vi "VersaLaseGUI_ForMain.vi"() -> ()   [LabVIEW 2014]
uses:
  C:/Users/Avogadro/Desktop/VersaUSB/VersaUSB.dll
  VersaUSB.dll
panel:
  out "ne":i32
  out "e":i32
  in  "Blu Pow":dbl(slide) scale=0.0..100.0
  in  "Grn Pow":dbl(slide) scale=0.0..40.0
  in  "Blu On":bool
  in  "Grn On":bool
  out "Blu Temp":dbl
  out "Grn Temp":dbl
  in  "Red Pow":dbl(slide) scale=0.0..100.0
  in  "Red On":bool
  out "Red Temp":dbl
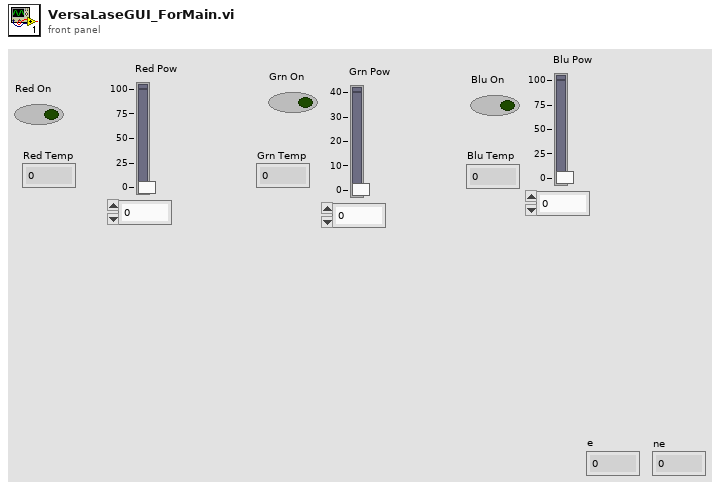
[diagram p1: front panel]
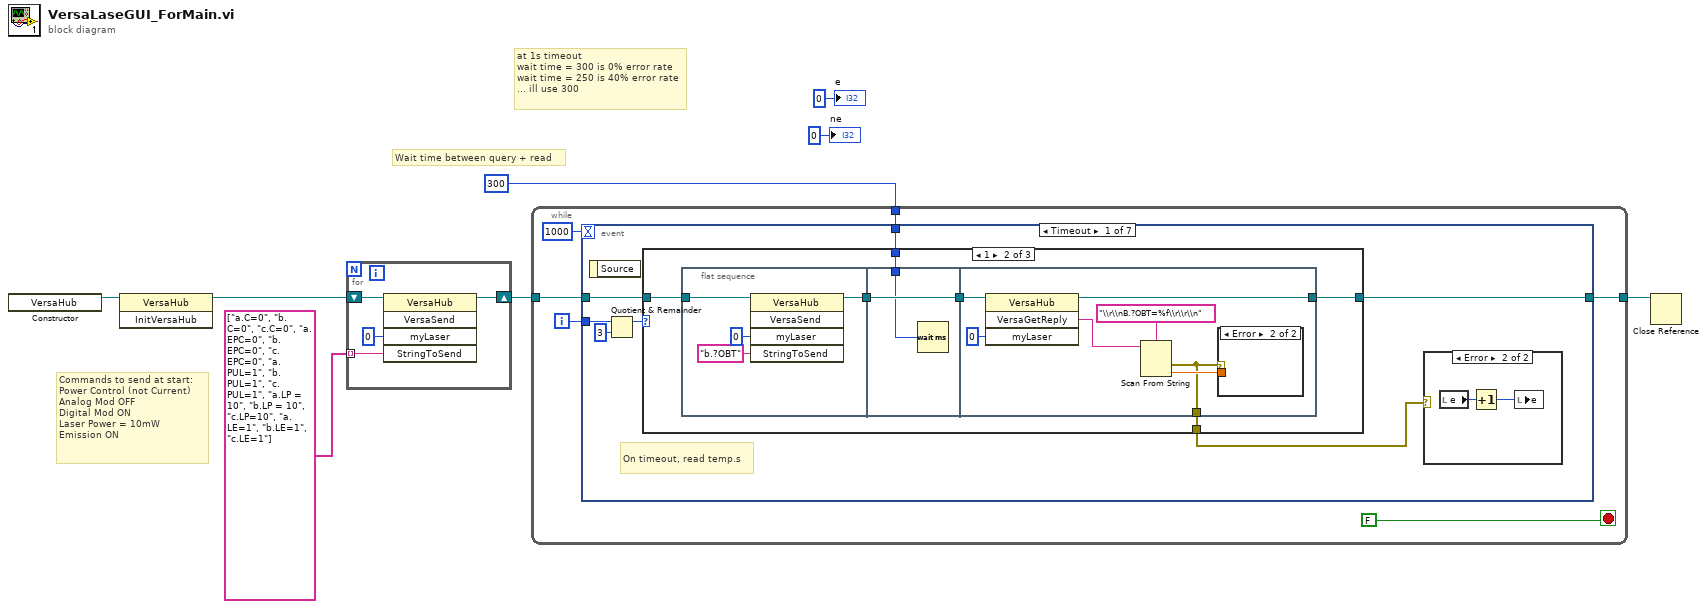
[diagram p0: block diagram]
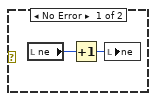
[diagram p2: hidden frame]
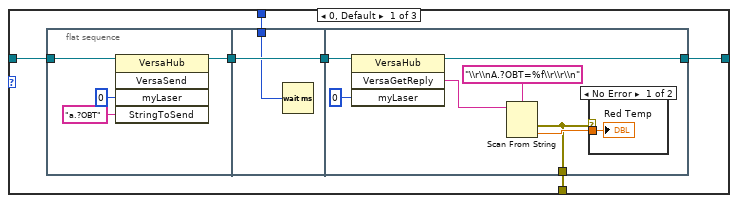
[diagram p3: hidden frame]
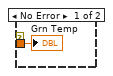
[diagram p5: hidden frame]
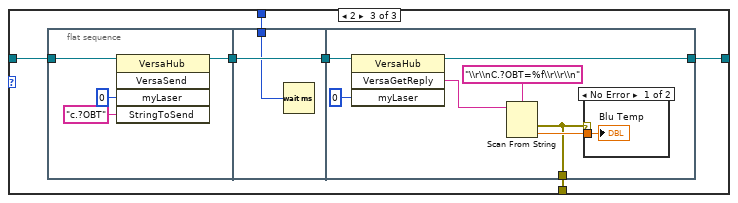
[diagram p6: hidden frame]
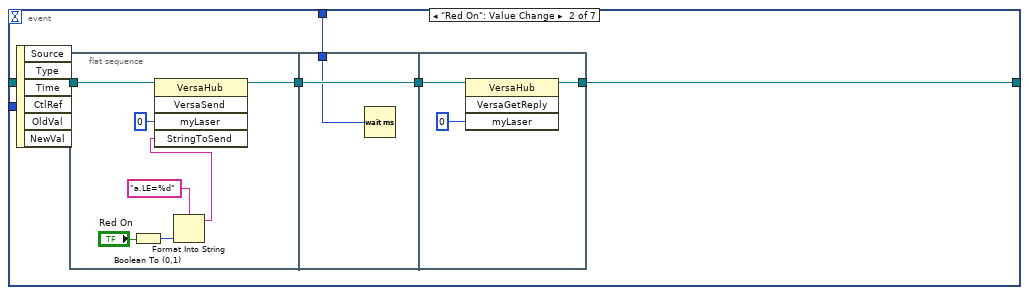
[diagram p8: hidden frame]
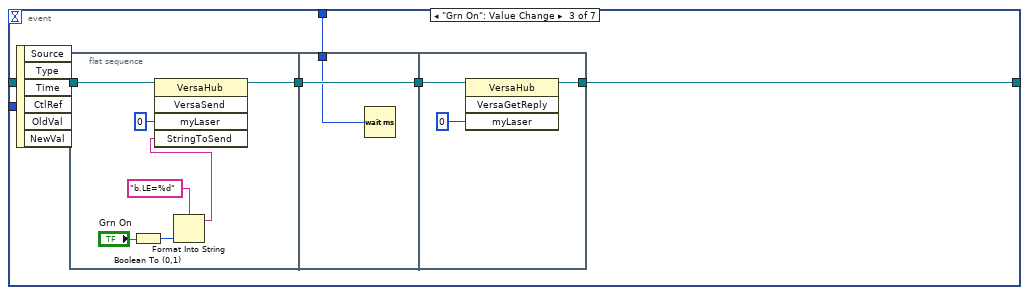
[diagram p9: hidden frame]
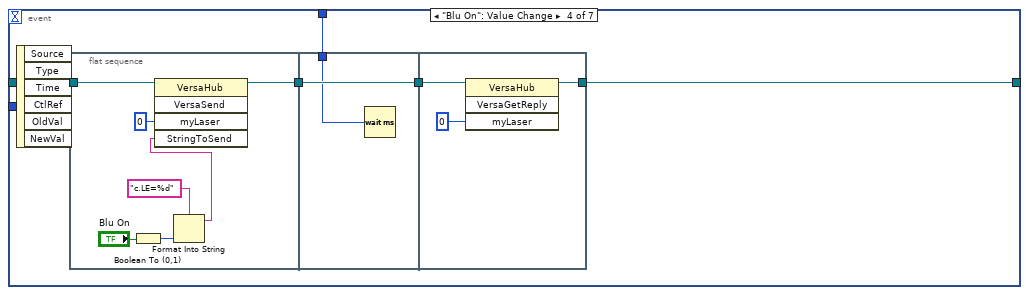
[diagram p10: hidden frame]
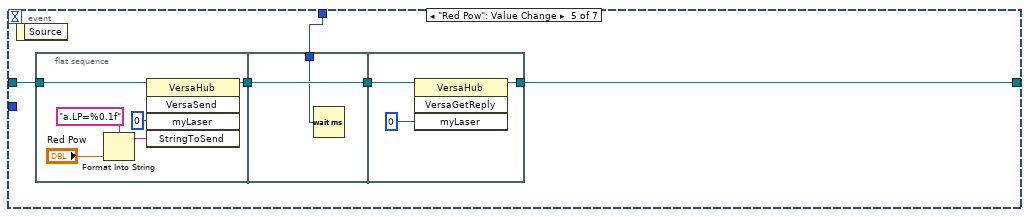
[diagram p11: hidden frame]
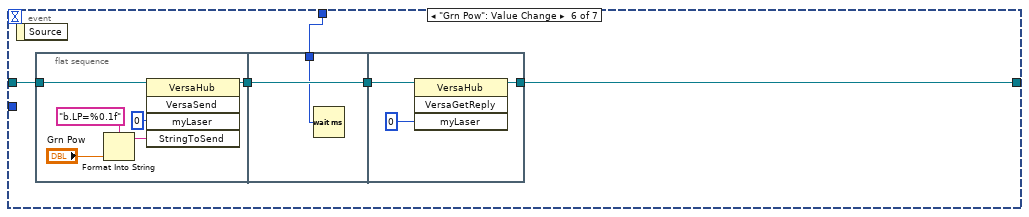
[diagram p12: hidden frame]
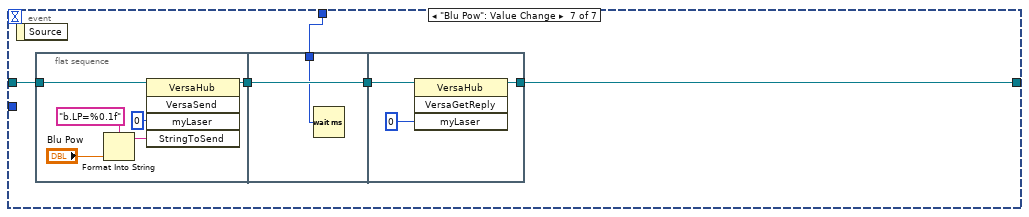
[diagram p13: hidden frame]
diagram:
  # "Wait time between query + read"
  # "Commands to send at start:\nPower Control (not Current)\nAnalog Mod OFF\nDigital Mod ON\nLaser Power = 10mW\nEmission ON"
  # "at 1s timeout\nwait time = 300 is 0% error rate\nwait time = 250 is 40% error rate\n... ill use 300"
  n1 = constructor class="VersaHub"() -> (reference out=w8:refnum<k24>)  [unwired: 3 in, 2 out]
  n2 = invoke class="VersaHub" method="InitVersaHub"(reference=w8) -> (reference out=w1:refnum<k24>)  [unwired: 2 in, 2 out]
  n3 = for {
    tunnel: string[] ["a.C=0", "b.C=0", "c.C=0", "a.EPC=0", "b.EPC=0", "c.EPC=0", "a.PUL=1", "b.PUL=1", "c.PUL=1", "a.LP = 10", "b.LP = 10", "c.LP=10", "a.LE=1", "b.LE=1", "c.LE=1"] -> [w11] mode=indexing
    shift-right: [w10] -> w2
    shift-left: w1 -> [w9]
    n4 = invoke class="VersaHub" method="VersaSend"(reference=w9, "myLaser"=0 ("moduleId"), "StringToSend"=w11) -> (reference out=w10:refnum<k24>)  [unwired: 2 in, 4 out]
  }
  n5 = while {
    tunnel: w2 -> [w18]
    tunnel: [w17] -> w7
    tunnel: u32 300 -> [w13]
    i -> [w14]
    stop <- FALSE stop-if-true
    n6 = event shown="[0] Timeout" {
      selector: _ -> [_ _ _ _ _ _ _]
      dyn-events: _ -> [_ _ _ _ _ _ _]
      timeout: 1000 -> [_ _ _ _ _ _ _]
      tunnel: w18 -> [w25 w94 w111 w128 w143 w159 w175]
      tunnel: [w19 w91 w108 w125 w142 w158 w174] -> w17
      tunnel: w14 -> [w24 _ _ _ _ _ _]
      tunnel: w13 -> [w21 w90 w107 w124 w141 w157 w173]
      event Timeout {
        # "On timeout, read temp.s"
        n7 = event-data() -> ()  [unwired: 1 in, 1 out]
        n8 = Quotient & Remainder(x=w24, y=3) -> (x-y*floor(x/y)=w23:i32)  [unwired: 1 out]
        n9 = case shown="1" w23 {
          tunnel: w25 -> [w33 w53 w73]
          tunnel: [w32 w52 w72] -> w19
          tunnel: w21 -> [w31 w51 w71]
          tunnel: [w30 w50 w70] -> w20
          frame 0, Default {
            n10 = flat-sequence {
              tunnel: w33 -> [w39]
              tunnel: [w36] -> w35
              tunnel: w35 -> [w41]
              tunnel: [w41] -> w34
              tunnel: w31 -> [w40]
              tunnel: [w43] -> w32
              tunnel: w34 -> [w47]
              tunnel: [w42] -> w30
              frame #0 {
                n11 = invoke class="VersaHub" method="VersaSend"(reference=w39, "myLaser"=0, "StringToSend"="a.?OBT") -> (reference out=w36:refnum<k24>)  [unwired: 2 in, 4 out]
              }
              frame #1 {
                n12 = Wait (ms)(milliseconds to wait=w40) -> ()  [unwired: 1 out]
              }
              frame #2 {
                n13 = invoke class="VersaHub" method="VersaGetReply"(reference=w47, "myLaser"=0) -> (reference out=w43:refnum<k24>, "VersaGetReply"=w44:string)  [unwired: 2 in, 2 out]
                n14 = Scan From String(format string="\\r\\nA.?OBT=%f\\r\\r\\n", input string=w44) -> (error out=w42:errorcluster, output 1=w45:dbl)  [unwired: 3 in, 2 out]
                n15 = case shown="No Error" w42 {
                  tunnel: w45 -> [w49 _]
                  frame No Error {
                    "Red Temp" <- w49
                  }
                  frame Error {
                  }
                }
              }
            }
          }
          frame 1 {
            n16 = flat-sequence {
              tunnel: w53 -> [w59]
              tunnel: [w56] -> w55
              tunnel: w55 -> [w61]
              tunnel: [w61] -> w54
              tunnel: w51 -> [w60]
              tunnel: [w63] -> w52
              tunnel: w54 -> [w67]
              tunnel: [w62] -> w50
              frame #0 {
                n17 = invoke class="VersaHub" method="VersaSend"(reference=w59, "myLaser"=0, "StringToSend"="b.?OBT") -> (reference out=w56:refnum<k24>)  [unwired: 2 in, 4 out]
              }
              frame #1 {
                n18 = Wait (ms)(milliseconds to wait=w60) -> ()  [unwired: 1 out]
              }
              frame #2 {
                n19 = invoke class="VersaHub" method="VersaGetReply"(reference=w67, "myLaser"=0) -> (reference out=w63:refnum<k24>, "VersaGetReply"=w64:string)  [unwired: 2 in, 2 out]
                n20 = Scan From String(format string="\\r\\nB.?OBT=%f\\r\\r\\n", input string=w64) -> (error out=w62:errorcluster, output 1=w65:dbl)  [unwired: 3 in, 2 out]
                n21 = case shown="Error" w62 {
                  tunnel: w65 -> [w69 _]
                  frame No Error {
                    "Grn Temp" <- w69
                  }
                  frame Error {
                  }
                }
              }
            }
          }
          frame 2 {
            n22 = flat-sequence {
              tunnel: w73 -> [w79]
              tunnel: [w76] -> w75
              tunnel: w75 -> [w81]
              tunnel: [w81] -> w74
              tunnel: w71 -> [w80]
              tunnel: [w83] -> w72
              tunnel: w74 -> [w87]
              tunnel: [w82] -> w70
              frame #0 {
                n23 = invoke class="VersaHub" method="VersaSend"(reference=w79, "myLaser"=0, "StringToSend"="c.?OBT") -> (reference out=w76:refnum<k24>)  [unwired: 2 in, 4 out]
              }
              frame #1 {
                n24 = Wait (ms)(milliseconds to wait=w80) -> ()  [unwired: 1 out]
              }
              frame #2 {
                n25 = invoke class="VersaHub" method="VersaGetReply"(reference=w87, "myLaser"=0) -> (reference out=w83:refnum<k24>, "VersaGetReply"=w84:string)  [unwired: 2 in, 2 out]
                n26 = Scan From String(format string="\\r\\nC.?OBT=%f\\r\\r\\n", input string=w84) -> (error out=w82:errorcluster, output 1=w85:dbl)  [unwired: 3 in, 2 out]
                n27 = case shown="No Error" w82 {
                  tunnel: w85 -> [w89 _]
                  frame No Error {
                    "Blu Temp" <- w89
                  }
                  frame Error {
                  }
                }
              }
            }
          }
        }
        n28 = case shown="Error" w20 {
          frame No Error {
            n29 = local read "ne"() -> (w27:i32)
            n30 = Increment(x=w27) -> (x+1=w26:i32)
            n31 = local write "ne"(w26) -> ()
          }
          frame Error {
            n32 = local read "e"() -> (w28:i32)
            n33 = Increment(x=w28) -> (x+1=w29:i32)
            n34 = local write "e"(w29) -> ()
          }
        }
      }
      event "Red On": Value Change {
        n35 = event-data() -> ()  [unwired: 1 in, 6 out]
        n36 = flat-sequence {
          tunnel: w94 -> [w101]
          tunnel: [w99] -> w93
          tunnel: w93 -> [w103]
          tunnel: [w103] -> w92
          tunnel: w90 -> [w102]
          tunnel: [w104] -> w91
          tunnel: w92 -> [w105]
          frame #0 {
            n37 = Boolean To (0,1)(Boolean="Red On") -> (0, 1=w97:i16)
            n38 = Format Into String(format string="a.LE=%d", w97) -> (resulting string=w95:string)  [unwired: 2 in, 1 out]
            n39 = invoke class="VersaHub" method="VersaSend"(reference=w101, "myLaser"=0, "StringToSend"=w95) -> (reference out=w99:refnum<k24>)  [unwired: 2 in, 4 out]
          }
          frame #1 {
            n40 = Wait (ms)(milliseconds to wait=w102) -> ()  [unwired: 1 out]
          }
          frame #2 {
            n41 = invoke class="VersaHub" method="VersaGetReply"(reference=w105, "myLaser"=0) -> (reference out=w104:refnum<k24>)  [unwired: 2 in, 3 out]
          }
        }
      }
      event "Grn On": Value Change {
        n42 = event-data() -> ()  [unwired: 1 in, 6 out]
        n43 = flat-sequence {
          tunnel: w111 -> [w118]
          tunnel: [w116] -> w110
          tunnel: w110 -> [w120]
          tunnel: [w120] -> w109
          tunnel: w107 -> [w119]
          tunnel: [w121] -> w108
          tunnel: w109 -> [w122]
          frame #0 {
            n44 = Boolean To (0,1)(Boolean="Grn On") -> (0, 1=w114:i16)
            n45 = Format Into String(format string="b.LE=%d", w114) -> (resulting string=w112:string)  [unwired: 2 in, 1 out]
            n46 = invoke class="VersaHub" method="VersaSend"(reference=w118, "myLaser"=0, "StringToSend"=w112) -> (reference out=w116:refnum<k24>)  [unwired: 2 in, 4 out]
          }
          frame #1 {
            n47 = Wait (ms)(milliseconds to wait=w119) -> ()  [unwired: 1 out]
          }
          frame #2 {
            n48 = invoke class="VersaHub" method="VersaGetReply"(reference=w122, "myLaser"=0) -> (reference out=w121:refnum<k24>)  [unwired: 2 in, 3 out]
          }
        }
      }
      event "Blu On": Value Change {
        n49 = event-data() -> ()  [unwired: 1 in, 6 out]
        n50 = flat-sequence {
          tunnel: w128 -> [w135]
          tunnel: [w133] -> w127
          tunnel: w127 -> [w137]
          tunnel: [w137] -> w126
          tunnel: w124 -> [w136]
          tunnel: [w138] -> w125
          tunnel: w126 -> [w139]
          frame #0 {
            n51 = Boolean To (0,1)(Boolean="Blu On") -> (0, 1=w131:i16)
            n52 = Format Into String(format string="c.LE=%d", w131) -> (resulting string=w129:string)  [unwired: 2 in, 1 out]
            n53 = invoke class="VersaHub" method="VersaSend"(reference=w135, "myLaser"=0, "StringToSend"=w129) -> (reference out=w133:refnum<k24>)  [unwired: 2 in, 4 out]
          }
          frame #1 {
            n54 = Wait (ms)(milliseconds to wait=w136) -> ()  [unwired: 1 out]
          }
          frame #2 {
            n55 = invoke class="VersaHub" method="VersaGetReply"(reference=w139, "myLaser"=0) -> (reference out=w138:refnum<k24>)  [unwired: 2 in, 3 out]
          }
        }
      }
      event "Red Pow": Value Change {
        n56 = event-data() -> ()  [unwired: 1 in, 1 out]
        n57 = flat-sequence {
          tunnel: w143 -> [w151]
          tunnel: [w149] -> w145
          tunnel: w145 -> [w153]
          tunnel: [w153] -> w144
          tunnel: w141 -> [w152]
          tunnel: [w154] -> w142
          tunnel: w144 -> [w155]
          frame #0 {
            n58 = Format Into String(format string="a.LP=%0.1f", "Red Pow") -> (resulting string=w146:string)  [unwired: 2 in, 1 out]
            n59 = invoke class="VersaHub" method="VersaSend"(reference=w151, "myLaser"=0, "StringToSend"=w146) -> (reference out=w149:refnum<k24>)  [unwired: 2 in, 4 out]
          }
          frame #1 {
            n60 = Wait (ms)(milliseconds to wait=w152) -> ()  [unwired: 1 out]
          }
          frame #2 {
            n61 = invoke class="VersaHub" method="VersaGetReply"(reference=w155, "myLaser"=0) -> (reference out=w154:refnum<k24>)  [unwired: 2 in, 3 out]
          }
        }
      }
      event "Grn Pow": Value Change {
        n62 = event-data() -> ()  [unwired: 1 in, 1 out]
        n63 = flat-sequence {
          tunnel: w159 -> [w167]
          tunnel: [w165] -> w161
          tunnel: w161 -> [w169]
          tunnel: [w169] -> w160
          tunnel: w157 -> [w168]
          tunnel: [w170] -> w158
          tunnel: w160 -> [w171]
          frame #0 {
            n64 = Format Into String(format string="b.LP=%0.1f", "Grn Pow") -> (resulting string=w162:string)  [unwired: 2 in, 1 out]
            n65 = invoke class="VersaHub" method="VersaSend"(reference=w167, "myLaser"=0, "StringToSend"=w162) -> (reference out=w165:refnum<k24>)  [unwired: 2 in, 4 out]
          }
          frame #1 {
            n66 = Wait (ms)(milliseconds to wait=w168) -> ()  [unwired: 1 out]
          }
          frame #2 {
            n67 = invoke class="VersaHub" method="VersaGetReply"(reference=w171, "myLaser"=0) -> (reference out=w170:refnum<k24>)  [unwired: 2 in, 3 out]
          }
        }
      }
      event "Blu Pow": Value Change {
        n68 = event-data() -> ()  [unwired: 1 in, 1 out]
        n69 = flat-sequence {
          tunnel: w175 -> [w183]
          tunnel: [w181] -> w177
          tunnel: w177 -> [w185]
          tunnel: [w185] -> w176
          tunnel: w173 -> [w184]
          tunnel: [w186] -> w174
          tunnel: w176 -> [w187]
          frame #0 {
            n70 = Format Into String(format string="b.LP=%0.1f", "Blu Pow") -> (resulting string=w178:string)  [unwired: 2 in, 1 out]
            n71 = invoke class="VersaHub" method="VersaSend"(reference=w183, "myLaser"=0, "StringToSend"=w178) -> (reference out=w181:refnum<k24>)  [unwired: 2 in, 4 out]
          }
          frame #1 {
            n72 = Wait (ms)(milliseconds to wait=w184) -> ()  [unwired: 1 out]
          }
          frame #2 {
            n73 = invoke class="VersaHub" method="VersaGetReply"(reference=w187, "myLaser"=0) -> (reference out=w186:refnum<k24>)  [unwired: 2 in, 3 out]
          }
        }
      }
    }
  }
  n74 = Close Reference(reference=w7) -> ()  [unwired: 1 in, 1 out]
  "e" <- 0 ("e")
  "ne" <- 0 ("ne")
